vi "Working_Test_Formatting.vi"() -> ()   [LabVIEW 2014]
doc: "This example shows how to read and write simple user events from and to a USB RAW device. \n\n<b>Note:</b> This example works only with USB RAW devices.\n\nBefore you run this VI, install a USB RAW device and configure NI Measurement & Automation Explorer (MAX) to recognize the USB device. You can read to and write from the USB RAW device only after you install and configure the USB RAW device and open a session to the device. To read to or write from another device, close the session to the current device, select another device from the <b>VISA Resource</b> control, and open a session to the new device. \n\nWhen you complete the read or write, click the <b>Stop</b> button to stop the VI."
panel:
  out "String":string
  in  "Numeric 25":dbl caption="Numeric 10" min=0.0 max=1000.0
  in  "Numeric 24":dbl caption="Numeric 10" min=0.0 max=100.0
  in  "Numeric 23":dbl caption="Numeric 10" min=0.0 max=6.0
  in  "Boolean 8":bool caption="Channel 7"
  in  "Numeric 22":dbl caption="Numeric 10" min=0.0 max=1000.0
  in  "Numeric 21":dbl caption="Numeric 10" min=0.0 max=100.0
  in  "Numeric 20":dbl caption="Numeric 10" min=0.0 max=6.0
  in  "Boolean 7":bool caption="Channel 6"
  in  "Numeric 19":dbl caption="Numeric 10" min=0.0 max=1000.0
  in  "Numeric 18":dbl caption="Numeric 10" min=0.0 max=100.0
  in  "Numeric 17":dbl caption="Numeric 10" min=0.0 max=6.0
  in  "Boolean 6":bool caption="Channel 5"
  in  "Numeric 16":dbl caption="Numeric 12" min=0.0 max=1000.0
  in  "Numeric 15":dbl caption="Numeric 11" min=0.0 max=100.0
  in  "Numeric 14":dbl caption="Numeric 10" min=0.0 max=6.0
  in  "Boolean 5":bool caption="Channel 4"
  in  "Start":bool caption="stop"
  in  "Boolean 4":bool caption="Channel 3"
  in  "Boolean 3":bool caption="Channel 2"
  in  "Boolean 2":bool caption="Channel 1"
  in  "Boolean":bool caption="Channel 0"
  in  "Numeric 13":dbl caption="Numeric 12" min=0.0 max=1000.0
  in  "Numeric 12":dbl caption="Numeric 11" min=0.0 max=100.0
  in  "Numeric 11":dbl caption="Numeric 10" min=0.0 max=6.0
  in  "Numeric 10":dbl caption="Numeric 9" min=0.0 max=1000.0
  in  "Numeric 9":dbl caption="Numeric 8" min=0.0 max=100.0
  in  "Numeric 8":dbl caption="Numeric 7" min=0.0 max=6.0
  in  "Numeric 7":dbl caption="Numeric 6" min=0.0 max=1000.0
  in  "Numeric 6":dbl caption="Numeric 5" min=0.0 max=100.0
  in  "Numeric 5":dbl caption="Numeric 4" min=0.0 max=6.0
  in  "Numeric 4":dbl caption="Numeric 3" min=0.0 max=1000.0
  in  "Numeric 3":dbl caption="Numeric 2" min=0.0 max=100.0
  in  "Numeric 2":dbl caption="Numeric" min=0.0 max=6.0
  out "Numeric":i32
  out "Waveform Chart":i32(graph)
  in  "?":string="The specified VISA resource is not a USB device."
  out "Bulk Read Response":string
  in  "Stop":bool
  in  "VISA Resource":refnum<visa-resource-name>
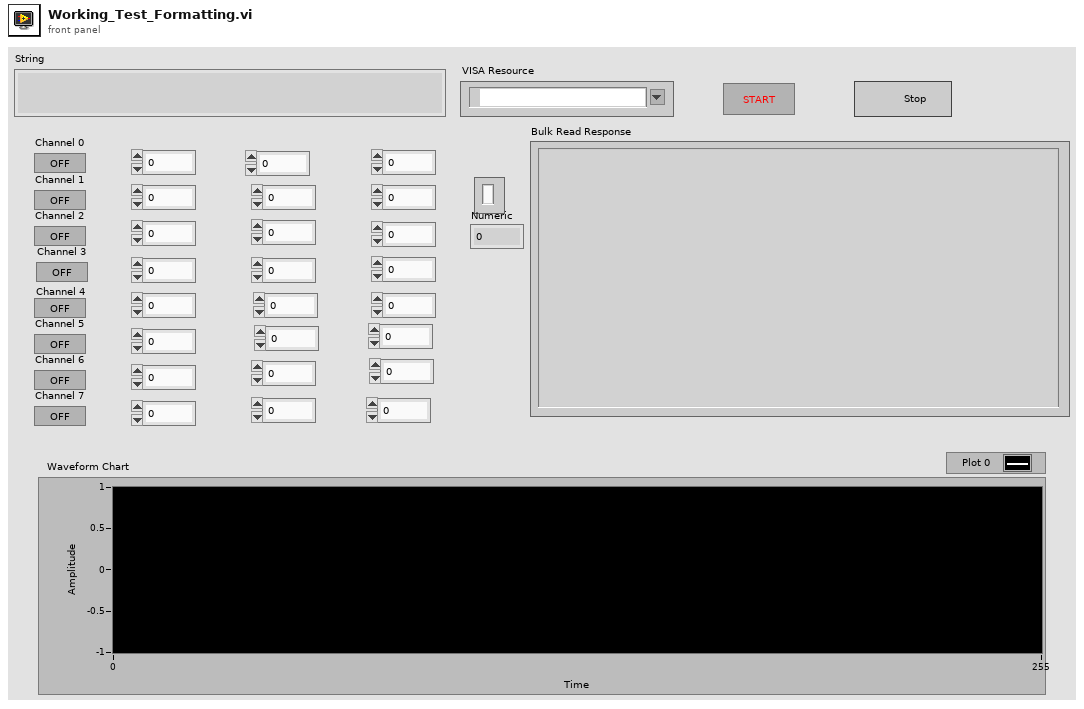
[diagram p1: front panel]
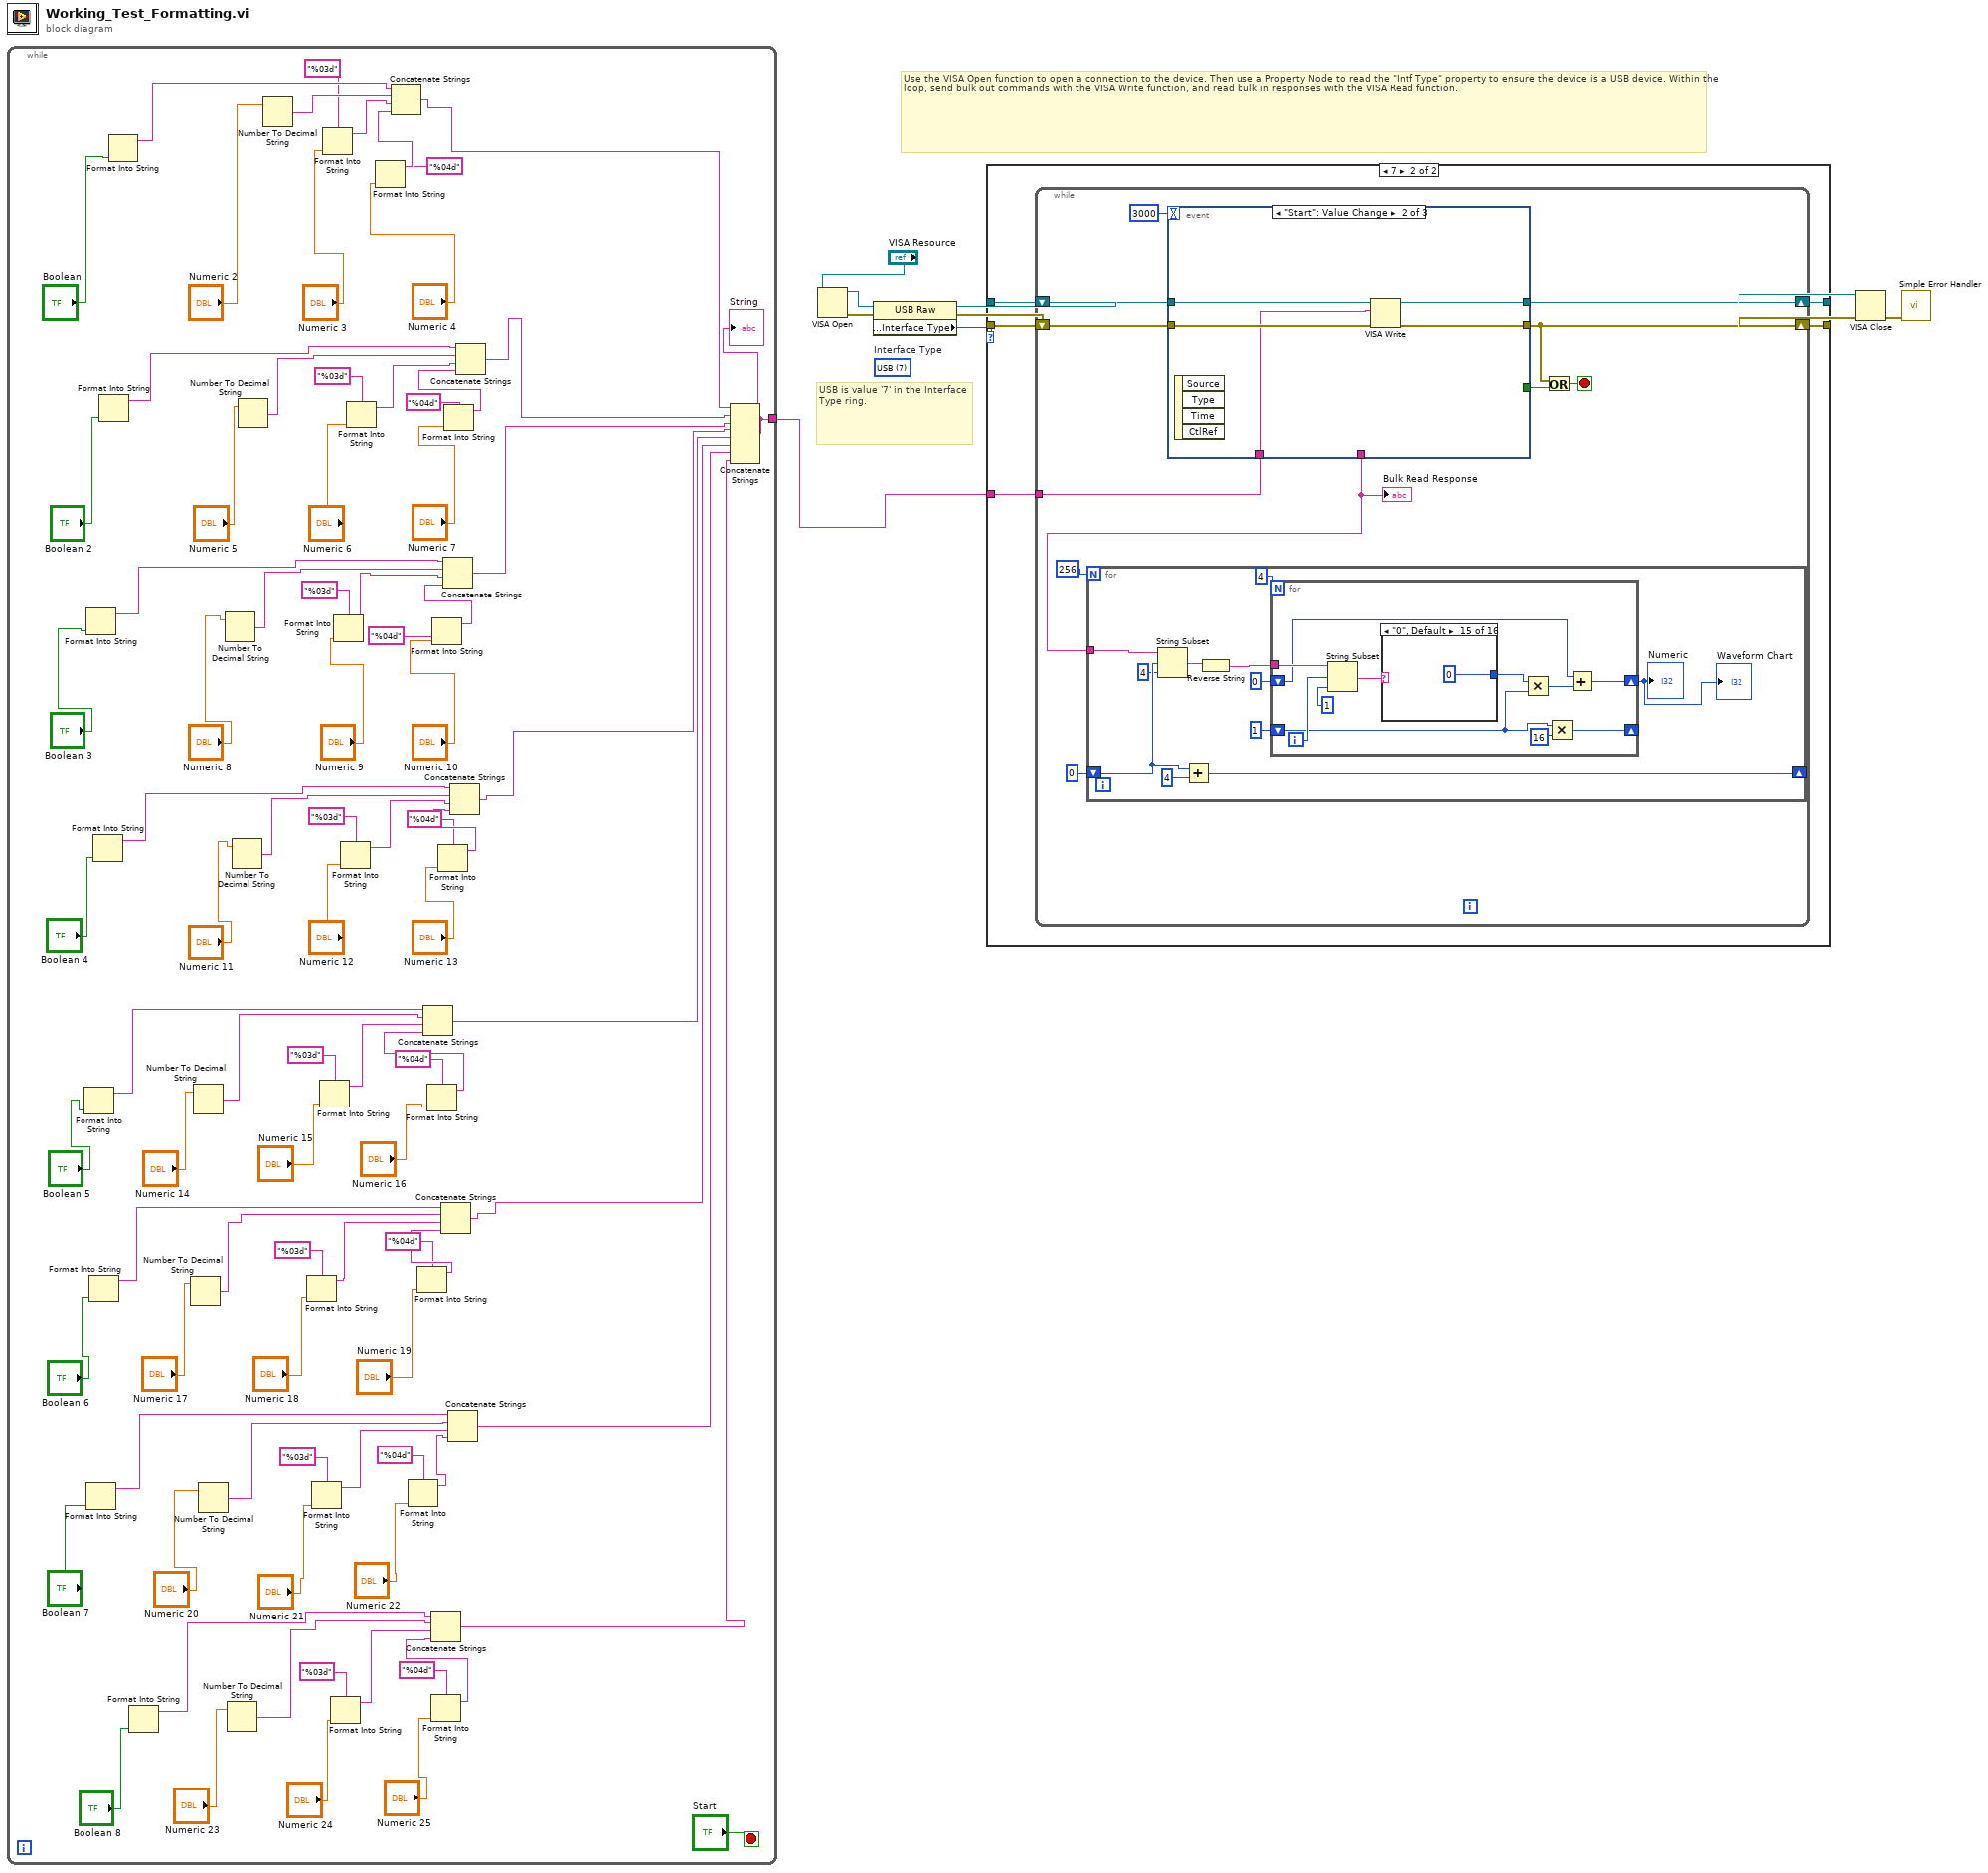
[diagram p0: block diagram]
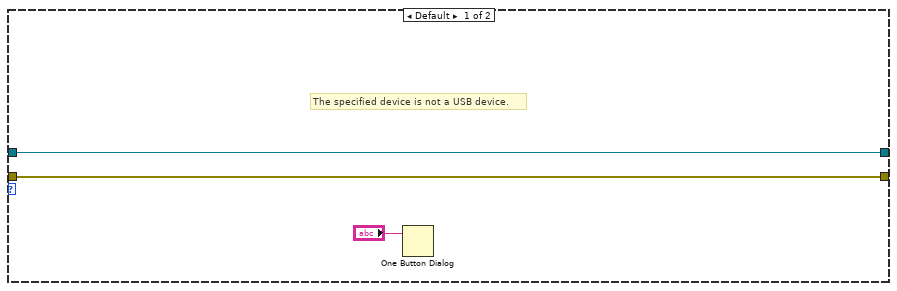
[diagram p2: hidden frame]
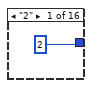
[diagram p3: hidden frame]
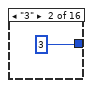
[diagram p4: hidden frame]
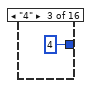
[diagram p5: hidden frame]
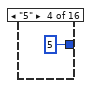
[diagram p6: hidden frame]
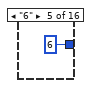
[diagram p7: hidden frame]
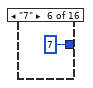
[diagram p8: hidden frame]
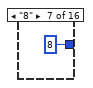
[diagram p9: hidden frame]
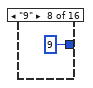
[diagram p10: hidden frame]
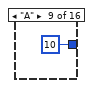
[diagram p11: hidden frame]
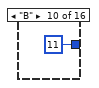
[diagram p12: hidden frame]
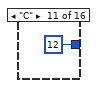
[diagram p13: hidden frame]
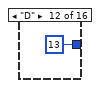
[diagram p14: hidden frame]
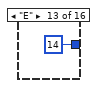
[diagram p15: hidden frame]
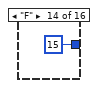
[diagram p16: hidden frame]
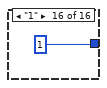
[diagram p17: hidden frame]
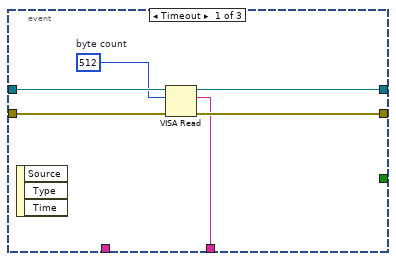
[diagram p18: hidden frame]
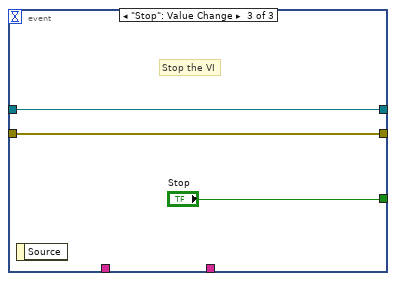
[diagram p19: hidden frame]
diagram:
  (unwired) u16 7 items=["GPIB"=1, "VXI"=2, "GPIB-VXI"=3, "Serial"=4, "PXI"=5, "TCPIP"=6, "USB"=7, "FireWire"=9]  # Interface Type
  # "Use the VISA Open function to open a connection to the device. Then use a Property Node to read the \"Intf Type\" property to ensure the device is a USB device. Within the loop, send bulk out commands with the VISA Write function, and read bulk in responses with the VISA Read function."
  # "USB is value '7' in the Interface Type ring."
  n1 = while {
    tunnel: [w62] -> w1
    stop <- "Start" stop-if-true
    n2 = Format Into String("Boolean 5") -> (resulting string=w81:string)  [unwired: 3 in, 1 out]
    n3 = Format Into String("Boolean 3") -> (resulting string=w94:string)  [unwired: 3 in, 1 out]
    n4 = Format Into String("Boolean 7") -> (resulting string=w72:string)  [unwired: 3 in, 1 out]
    n5 = Format Into String("Boolean 6") -> (resulting string=w75:string)  [unwired: 3 in, 1 out]
    n6 = Format Into String("Boolean 4") -> (resulting string=w90:string)  [unwired: 3 in, 1 out]
    n7 = Format Into String("Boolean 2") -> (resulting string=w96:string)  [unwired: 3 in, 1 out]
    n8 = Format Into String("Boolean") -> (resulting string=w99:string)  [unwired: 3 in, 1 out]
    n9 = Format Into String("Boolean 8") -> (resulting string=w69:string)  [unwired: 3 in, 1 out]
    n10 = Number To Decimal String(number="Numeric 17") -> (decimal integer string=w76:string)  [unwired: 1 in]
    n11 = Number To Decimal String(number="Numeric 14") -> (decimal integer string=w79:string)  [unwired: 1 in]
    n12 = Number To Decimal String(number="Numeric 20") -> (decimal integer string=w71:string)  [unwired: 1 in]
    n13 = Number To Decimal String(number="Numeric 8") -> (decimal integer string=w93:string)  [unwired: 1 in]
    n14 = Number To Decimal String(number="Numeric 23") -> (decimal integer string=w68:string)  [unwired: 1 in]
    n15 = Number To Decimal String(number="Numeric 11") -> (decimal integer string=w89:string)  [unwired: 1 in]
    n16 = Number To Decimal String(number="Numeric 5") -> (decimal integer string=w95:string)  [unwired: 1 in]
    n17 = Number To Decimal String(number="Numeric 2") -> (decimal integer string=w60:string)  [unwired: 1 in]
    n18 = Format Into String(format string="%03d", "Numeric 18") -> (resulting string=w28:string)  [unwired: 2 in, 1 out]
    n19 = Format Into String(format string="%03d", "Numeric 21") -> (resulting string=w22:string)  [unwired: 2 in, 1 out]
    n20 = Format Into String(format string="%03d", "Numeric 15") -> (resulting string=w33:string)  [unwired: 2 in, 1 out]
    n21 = Format Into String(format string="%03d", "Numeric 3") -> (resulting string=w59:string)  [unwired: 2 in, 1 out]
    n22 = Format Into String(format string="%03d", "Numeric 24") -> (resulting string=w15:string)  [unwired: 2 in, 1 out]
    n23 = Format Into String(format string="%03d", "Numeric 9") -> (resulting string=w46:string)  [unwired: 2 in, 1 out]
    n24 = Format Into String(format string="%03d", "Numeric 12") -> (resulting string=w39:string)  [unwired: 2 in, 1 out]
    n25 = Format Into String(format string="%03d", "Numeric 6") -> (resulting string=w51:string)  [unwired: 2 in, 1 out]
    n26 = Format Into String(format string="%04d", "Numeric 4") -> (resulting string=w54:string)  [unwired: 2 in, 1 out]
    n27 = Concatenate Strings(w99, w60, w59, w54) -> (w86:string)
    n28 = Format Into String(format string="%04d", "Numeric 22") -> (resulting string=w19:string)  [unwired: 2 in, 1 out]
    n29 = Format Into String(format string="%04d", "Numeric 19") -> (resulting string=w25:string)  [unwired: 2 in, 1 out]
    n30 = Format Into String(format string="%04d", "Numeric 16") -> (resulting string=w31:string)  [unwired: 2 in, 1 out]
    n31 = Concatenate Strings(w81, w79, w33, w31) -> (w66:string)
    n32 = Format Into String(format string="%04d", "Numeric 25") -> (resulting string=w16:string)  [unwired: 2 in, 1 out]
    n33 = Concatenate Strings(w69, w68, w15, w16) -> (w63:string)
    n34 = Format Into String(format string="%04d", "Numeric 10") -> (resulting string=w41:string)  [unwired: 2 in, 1 out]
    n35 = Format Into String(format string="%04d", "Numeric 13") -> (resulting string=w38:string)  [unwired: 2 in, 1 out]
    n36 = Concatenate Strings(w75, w76, w28, w25) -> (w65:string)
    n37 = Concatenate Strings(w94, w93, w46, w41) -> (w84:string)
    n38 = Format Into String(format string="%04d", "Numeric 7") -> (resulting string=w48:string)  [unwired: 2 in, 1 out]
    n39 = Concatenate Strings(w72, w71, w22, w19) -> (w64:string)
    n40 = Concatenate Strings(w90, w89, w39, w38) -> (w83:string)
    n41 = Concatenate Strings(w96, w95, w51, w48) -> (w85:string)
    n42 = Concatenate Strings(w86, w85, w84, w83, w66, w65, w64, w63) -> (w62:string)
    "String" <- w62
  }
  n43 = VISA Open(VISA resource name="VISA Resource") -> (VISA resource name=w9:refnum<visa-resource-name>, error out=w10:errorcluster)  [unwired: 1 in, 3 out]
  n44 = property class="USB Raw"(reference=w9, error in=w10) -> (reference out=w3:refnum<visa-resource-name>, error out=w4:errorcluster, "Interface Information:Interface Type"=w2:u16)
  n45 = case shown="7" w2 {
    tunnel: [w103 w108] -> w7
    tunnel: [w102 w107] -> w5
    tunnel: w4 -> [w103 w106]
    tunnel: w3 -> [w102 w105]
    tunnel: w1 -> [_ w104]
    frame Default {
      # "The specified device is not a USB device."
      n46 = One Button Dialog(message="?") -> ()  [unwired: 1 in, 1 out]
    }
    frame 7 {
      n47 = while {
        shift-right: [w115] -> w108
        shift-left: w106 -> [w114]
        shift-right: [w117] -> w107
        shift-left: w105 -> [w116]
        tunnel: w104 -> [w111]
        stop <- w118 stop-if-true
        n48 = event shown="[1] \"Start\": Value Change" {
          selector: _ -> [_ _ _]
          dyn-events: _ -> [_ _ _]
          timeout: 3000 -> [_ _ _]
          tunnel: [_ _ "Stop"] -> w119
          tunnel: [w163 w167 w169] -> w115
          tunnel: w114 -> [w161 w168 w169]
          tunnel: [w162 w166 w170] -> w117
          tunnel: w116 -> [w160 w165 w170]
          tunnel: [w158 _ _] -> w110
          tunnel: w111 -> [_ w164 _]
          event Timeout {
            w159 = u32 512  # byte count
            n49 = event-data() -> ()  [unwired: 4 out]
            n50 = VISA Read(VISA resource name=w160, byte count=w159, error in (no error)=w161) -> (VISA resource name out=w162:refnum<visa-resource-name>, read buffer=w158:string, error out=w163:errorcluster)  [unwired: 1 out]
          }
          event "Start": Value Change {
            n51 = event-data() -> ()  [unwired: 5 out]
            n52 = VISA Write(VISA resource name=w165, write buffer=w164, error in (no error)=w168) -> (VISA resource name out=w166:refnum<visa-resource-name>, error out=w167:errorcluster)  [unwired: 1 out]
          }
          event "Stop": Value Change {
            # "Stop the VI"
            n53 = event-data() -> ()  [unwired: 2 out]
          }
        }
        "Bulk Read Response" <- w110
        n54 = for {
          N: 256 -> [_]
          tunnel: w110 -> [w126]
          shift-right: [w124] -> _
          shift-left: 0 -> [w123]
          n55 = String Subset(string=w126, offset (0)=w123, length (rest)=4 ("length (rest)")) -> (substring=w121:string)
          n56 = Add(x=w123, y=4) -> (x+y=w124:i32)
          n57 = Reverse String(1:w121) -> (0:w130:string)
          n58 = for {
            N: 4 -> [_]
            tunnel: w130 -> [w141]
            shift-right: [w135] -> _
            shift-left: 1 -> [w134]
            shift-right: [w132] -> w120
            shift-left: 0 -> [w131]
            i -> [w140]
            n59 = String Subset(string=w141, offset (0)=w140, length (rest)=1 ("length (rest)")) -> (substring=w138:string)
            n60 = case shown="\"0\", Default" w138 {
              tunnel: [2 3 4 5 6 7 8 9 10 11 12 13 14 15 0 1] -> w137
              frame "2" {
              }
              frame "3" {
              }
              frame "4" {
              }
              frame "5" {
              }
              frame "6" {
              }
              frame "7" {
              }
              frame "8" {
              }
              frame "9" {
              }
              frame "A" {
              }
              frame "B" {
              }
              frame "C" {
              }
              frame "D" {
              }
              frame "E" {
              }
              frame "F" {
              }
              frame "0", Default {
              }
              frame "1" {
              }
            }
            n61 = Multiply(x=w137, y=w134) -> (x*y=w133:i32)
            n62 = Multiply(x=w134, y=16) -> (x*y=w135:i32)
            n63 = Add(x=w131, y=w133) -> (x+y=w132:i32)
          }
          "Numeric" <- w120
          "Waveform Chart" <- w120
        }
        n64 = Or(x=w115, y=w119) -> (x .or. y?=w118:bool)
      }
    }
  }
  n65 = VISA Close(VISA resource name=w5, error in (no error)=w7) -> (error out=w6:errorcluster)
  n66 = call <vilib>:"Simple Error Handler.vi"("error in (no error)"=w6) -> ()  [unwired: 1 in, 8 out]
